vi "H5Aread_AdaptToInputs.Element.vi"(3 "Term Types":T1[](array[typedef]), 4 "XRef":refnum<vi>, 5 "State In":T4) -> (0 "Reply":string[](array[string]), 2 "State Out":T4)   [LabVIEW 2017, in "H5Aread.xnode"]
uses:
  <vilib>/UPVI/lvhdf5/attribute.llb/H5Aread.xnode
  <vilib>/UPVI/lvhdf5/attribute.llb/H5Aread/H5Aread_State.ctl
  <vilib>/UPVI/lvhdf5/xnodehelpers/TermsPlus.ctl
  <vilib>/XNodeSupport/XNodeTerm3.ctl
  <vilib>/XNodeSupport/XNodeString.ctl
  <vilib>/XNodeSupport/XNodeVariant.ctl
  <vilib>/XNodeSupport/XNodeRect32.ctl
  <vilib>/XNodeSupport/XNodeInt.ctl
  <vilib>/XNodeSupport/XNodeBool.ctl
  <vilib>/XNodeSupport/XNodeTermDirection.ctl
  <vilib>/UPVI/lvhdf5/xnodehelpers/TermBehavior.ctl
  <vilib>/XNodeSupport/XNodeError3Array.ctl
  <vilib>/XNodeSupport/XNodeError3.ctl
  <vilib>/XNodeSupport/XNodeTermTypeIDPair.ctl
  <vilib>/XNodeSupport/XNodeType.ctl
  <vilib>/XNodeSupport/NI_XNodeSupport.lvlib
panel:
  # "LVHDF5 Toolkit\nCopyright (c) 2005-2013 by Jason D. Sommerville\nCopyright (c) 2014 by UPVI, LLC.\n\nThis use and distribution of this file is governed by the terms found in \nLICENSE.txt distributed with this toolkit and installed at\n <user.lib>\\_lvhdf5\\LICENSE.txt"
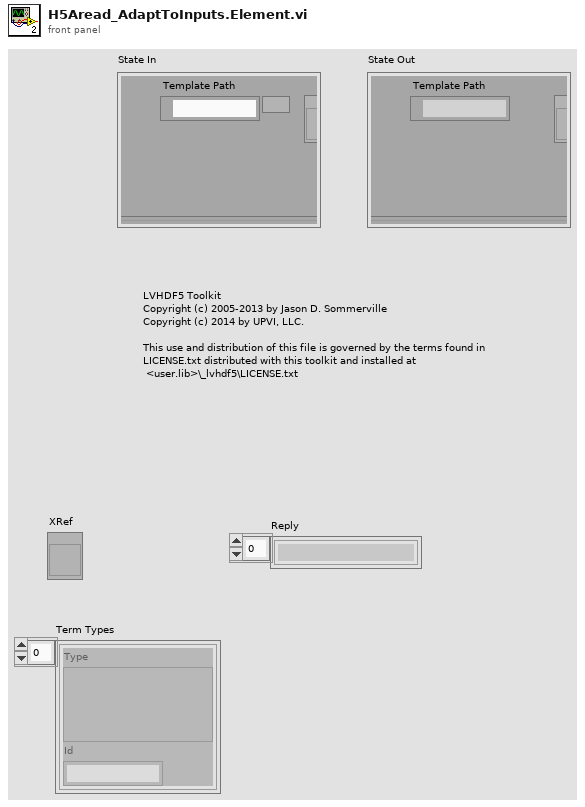
[diagram p1: front panel]
types:
  T1 = typedef "NI_XNodeSupport.lvlib/XNodeTermTypeIDPair.ctl" = cluster{"Type":T2, "Id":T3}
  T2 = typedef "NI_XNodeSupport.lvlib/XNodeType.ctl" = variant
  T3 = typedef "NI_XNodeSupport.lvlib/XNodeString.ctl" = string
  T4 = typedef "H5Aread.xnode/H5Aread_State.ctl" = cluster{"Template Path":path, "Template Ref":refnum<vi>, "Terms":T5[], "Display Name":string, "Image":picture, "Errors":T13, "Generated?":bool}
  T5 = typedef "TermsPlus.ctl" = cluster{"Term 3":T6, "Default Type":variant, "Behavior":T12, "Behavior Arg":string, "WiredResponse":bool, "Wired":enum16{"Unknown", "Unwired", "Wired"}}
  T6 = typedef "NI_XNodeSupport.lvlib/XNodeTerm3.ctl" = cluster{"Name":T3, "Id":T3, "Type":T7, "Bounds":T8, "Input?":T10, "Required?":T10, "Recommended?":T10, "Adaptive?":T10, "Hidden?":T10, "Direction":T11, "Break Wire?":T10}
  T7 = typedef "NI_XNodeSupport.lvlib/XNodeVariant.ctl" = variant
  T8 = typedef "NI_XNodeSupport.lvlib/XNodeRect32.ctl" = cluster{"Left":T9, "Top":T9, "Right":T9, "Bottom":T9}
  T9 = typedef "NI_XNodeSupport.lvlib/XNodeInt.ctl" = i32
  T10 = typedef "NI_XNodeSupport.lvlib/XNodeBool.ctl" = bool
  T11 = typedef "NI_XNodeSupport.lvlib/XNodeTermDirection.ctl" = enum32{"Auto", "Up", "Down", "Left", "Right", "Center"}
  T12 = typedef "TermBehavior.ctl" = enum16{"Normal", "Anything", "LVType", "Path or Ref", "Attr Name", "Attr Poly", "Elt Poly", "Dset Poly", "WDT Poly"}
  T13 = typedef "NI_XNodeSupport.lvlib/XNodeError3Array.ctl" = T14[]
  T14 = typedef "NI_XNodeSupport.lvlib/XNodeError3.ctl" = cluster{"Error":T3, "Details":T3, "Help File":T3, "Help Topic":T3}
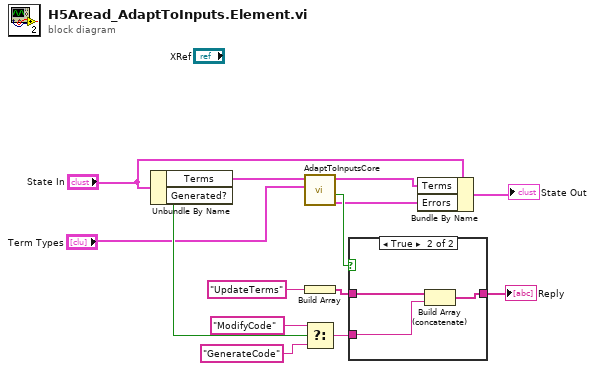
[diagram p0: block diagram]
diagram:
  n1 = Unbundle By Name("State In") -> ("Terms"=w8:T5[], "Generated?"=w9:bool)
  n2 = call <vilib>:"AdaptToInputsCore.vi"("Wired Terms"="Term Types", "Template Terms"=w8) -> ("Errors out"=w5:T14[], "Terms Modified?"=w6:bool, "Terms Out"=w7:T5[])  [unwired: 7 in]
  n3 = Build Array("UpdateTerms" ("String")) -> (w13:string[])
  n4 = Select(t="ModifyCode", s=w9, f="GenerateCode") -> (s? t:f=w10:string)
  n5 = case shown="True" w6 {
    tunnel: w13 -> [w15 w18]
    tunnel: [w15 w17] -> w2
    tunnel: w10 -> [_ w16]
    frame False {
    }
    frame True {
      n6 = Build Array (concatenate)(w18, w16) -> (w17:string[])
    }
  }
  "Reply" <- w2
  n7 = Bundle By Name(cluster="State In", "Terms"=w7, "Errors"=w5) -> (→"State Out":T4)
